vi "Inicializar_PWM (SubVI).vi"(8 "error in (no error)":errorcluster) -> (0 "error out":errorcluster, 1 "Esteira":T1, 2 "Atuador":T1, 3 "Elos do braço":T1[](array[typedef]))   [LabVIEW 2017]
uses:
  <vilib>/myRIO/Instrument Drivers/Onboard IO/PWM/typedefs/PWM Configuration.ctl
  <vilib>/myRIO/Instrument Drivers/Onboard IO/PWM/PWM.lvlib
  <vilib>/myRIO/Common/Instrument Driver Framework/myRIO v1.0/PWM/typedefs/PWM Channels Enum.ctl
  <vilib>/myRIO/Common/Instrument Driver Framework/Utilities/typedefs/Generic FPGA Reference.ctl
  <vilib>/myRIO/Common/Instrument Driver Framework/Utilities/typedefs/myRIO v1.0 Reference.ctl
  <vilib>/myRIO/Common/Instrument Driver Framework/Utilities/typedefs/Hardware Version Enum.ctl
  <vilib>/myRIO/Common/Instrument Driver Framework/Utilities/typedefs/myRIO Generic Hardware Reference.ctl
  <vilib>/myRIO/Instrument Drivers/Onboard IO/PWM/typedefs/PWM Reference.ctl
  <vilib>/userdefined/High Color/nirio_resource_hc.ctl
  <vilib>/myRIO/Common/Instrument Driver Framework/myRIO v1.0/PWM/vis/myRIO v1.1 Open PWM.vi
  <vilib>/myRIO/Instrument Drivers/Onboard IO/PWM/vis/myRIO PWM Open.xnode
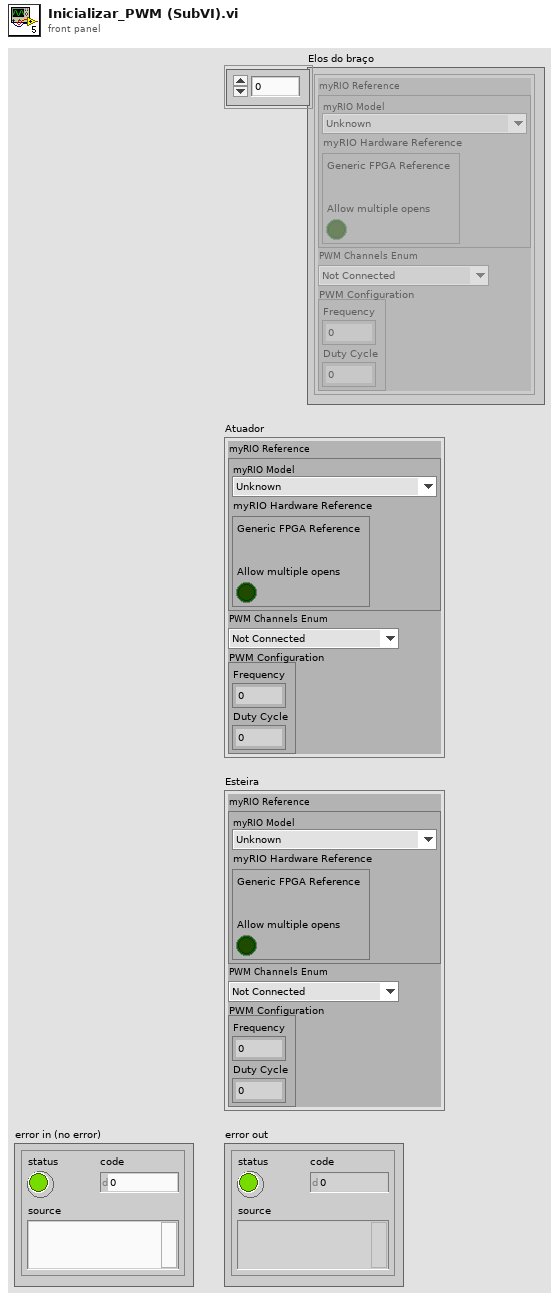
[diagram p1: front panel]
types:
  T1 = typedef "PWM.lvlib/PWM Reference.ctl" = cluster{"myRIO Reference":T2, "PWM Channels Enum":T6, "PWM Configuration":T7}
  T2 = typedef "myRIO Generic Hardware Reference.ctl" = cluster{"myRIO Model":T3, "myRIO Hardware Reference":T4}
  T3 = typedef "Hardware Version Enum.ctl" = enum16{"Unknown", "myRIO-1900", "myRIO-1950", "roboRIO", "NI ELVIS RIO CM"}
  T4 = typedef "myRIO v1.0 Reference.ctl" = cluster{"Generic FPGA Reference":T5, "Allow multiple opens":bool}
  T5 = typedef "Generic FPGA Reference.ctl" = refnum<k20>
  T6 = typedef "PWM Channels Enum.ctl" = enum16{"Not Connected", "C/PWM0", "C/PWM1", "A/PWM0", "A/PWM1", "A/PWM2", "B/PWM0", "B/PWM1", "B/PWM2", "PWM/PWM0", "PWM/PWM1", "PWM/PWM2", "PWM/PWM3", "PWM/PWM4", "PWM/PWM5", "PWM/PWM6", "PWM/PWM7", "PWM/PWM8", "PWM/PWM9"}
  T7 = typedef "PWM.lvlib/PWM Configuration.ctl" = cluster{"Frequency":dbl, "Duty Cycle":dbl}
  T8 = typedef "nirio_resource_hc.ctl" = tag
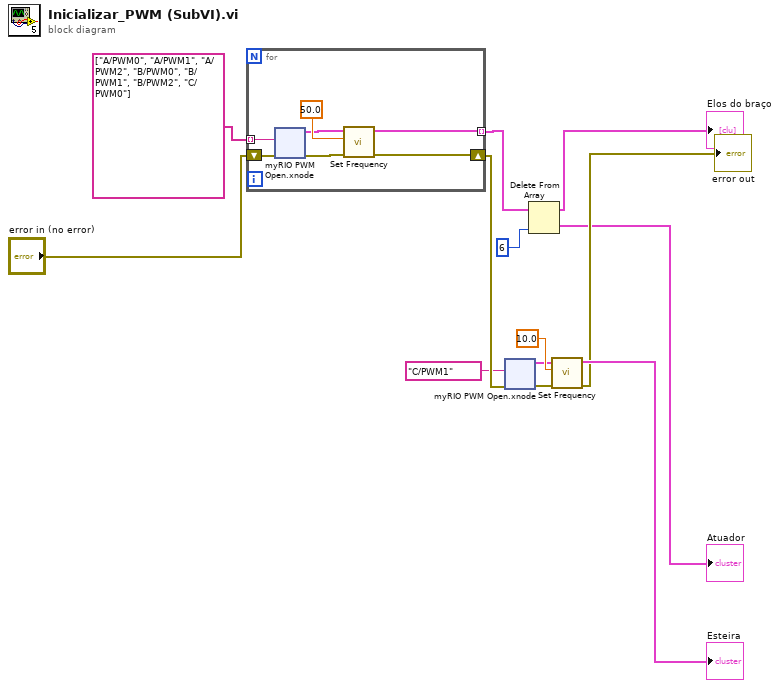
[diagram p0: block diagram]
diagram:
  n1 = for {
    shift-right: [w14] -> w8
    shift-left: "error in (no error)" -> [w19]
    tunnel: tag[] ["A/PWM0", "A/PWM1", "A/PWM2", "B/PWM0", "B/PWM1", "B/PWM2", "C/PWM0"] -> [w20] mode=indexing
    tunnel: [w15] -> w3 mode=indexing
    n2 = xnode "myRIO PWM Open.xnode"("error in (no error)"=w19, "Channel Name"=w20) -> ("error out"=w17:errorcluster, "PWM Ref Out"=w16:T1)  [unwired: 1 in]
    n3 = call <vilib>:"Set Frequency.vi"("error in (no error)"=w17, "Frequency [Hz]"=50.0, "PWM Ref In"=w16) -> ("error out"=w14:errorcluster, "PWM Ref Out"=w15:T1)  [unwired: 6 in]
  }
  n4 = xnode "myRIO PWM Open.xnode"("error in (no error)"=w8, "Channel Name"=tag "C/PWM1") -> ("error out"=w9:errorcluster, "PWM Ref Out"=w10:T1)  [unwired: 1 in]
  n5 = Delete From Array(array=w3, index=6) -> (deleted portion=→"Atuador":T1, array with subset deleted=→"Elos do braço":T1[])  [unwired: 1 in]
  n6 = call <vilib>:"Set Frequency.vi"("error in (no error)"=w9, "Frequency [Hz]"=10.0, "PWM Ref In"=w10) -> ("error out"=→"error out":errorcluster, "PWM Ref Out"=→"Esteira":T1)  [unwired: 6 in]
